vi "FTW-XML-Query-ElementValue.vi"(0 "XML Node":refnum<k20>, 5 "XPath":string, 11 "error in":errorcluster) -> (4 "XML Node out":refnum<k20>, 6 "Value":string, 8 "Found?":bool, 15 "error out":errorcluster)   [LabVIEW 2013]
uses:
  ftw-dataflow/Core/src/Error/FTW-ERR-ThrowError.vi
  <resource>/objmgr/DOMUserDefRef.rc
panel:
  # "Inputs"
  # "Outputs"
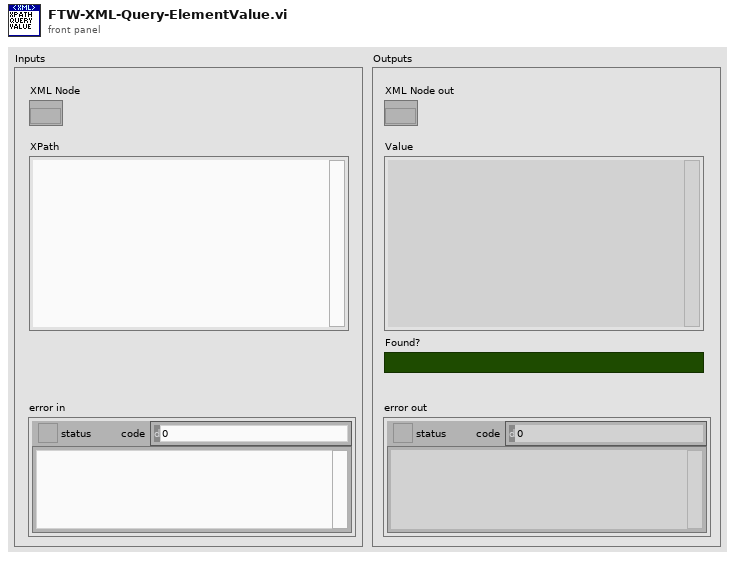
[diagram p1: front panel]
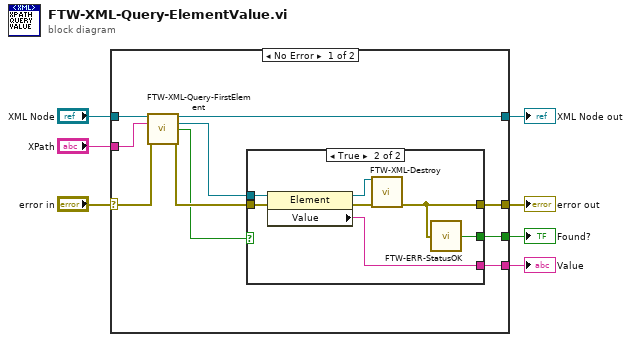
[diagram p0: block diagram]
diagram:
  n1 = case shown="No Error" "error in" {
    selector: "error in" -> [w11 w27]
    tunnel: [w17 w27] -> w7
    tunnel: "XML Node" -> [w13 w26]
    tunnel: [w14 w26] -> w4
    tunnel: "XPath" -> [w12 _]
    tunnel: [w16 _] -> w2
    tunnel: [w15 _] -> w1
    frame No Error {
      n2 = call "FTW-XML-Query-FirstElement.vi"("XML Node"=w13, "XPath Query"=w12, "error in"=w11) -> ("XML Node out"=w14:refnum<k20>, "First Matched Element"=w8:refnum<k20>, "Found?"=w9:bool, "error out"=w10:errorcluster)  [unwired: 8 in, 1 out]
      n3 = case shown="True" w9 {
        tunnel: w10 -> [w18 w25]
        tunnel: [w18 w19] -> w17
        tunnel: [_ w24] -> w16
        tunnel: w8 -> [_ w23]
        tunnel: [_ w22] -> w15
        frame False {
        }
        frame True {
          n4 = property class="Element"(reference=w23, error in=w25) -> (reference out=w21:refnum<k20>, error out=w20:errorcluster, "Value"=w24:string)
          n5 = call "FTW-XML-Destroy.vi"("XML Node"=w21, "error in"=w20) -> ("error out"=w19:errorcluster)  [unwired: 13 in]
          n6 = call "FTW-ERR-StatusOK.vi"("error to check"=w19) -> ("Status OK?"=w22:bool)
        }
      }
    }
    frame Error {
    }
  }
  "error out" <- w7
  "XML Node out" <- w4
  "Found?" <- w1
  "Value" <- w2
